vi "PWM Config.vi"(8 "error in (no error)":errorcluster, 11 "Config in":refnum<class "Config.lvclass">) -> (0 "error out":errorcluster, 1 "IDs found?":bool, 2 "PWM Data":T1, 3 "Config out":refnum<class "Config.lvclass">, 5 "File Found?":bool)   [LabVIEW 2019, in "Config.lvlib" / "Config.lvclass"]
doc: "Use this VI to retrieve the PWM channels that will be used in the robot."
uses:
  Config.lvclass
  Controls/PWM Data.ctl
  <vilib>/Rock Robotics/SystemInterfaces/DIO/FPGA_DIOPWMChannel.ctl
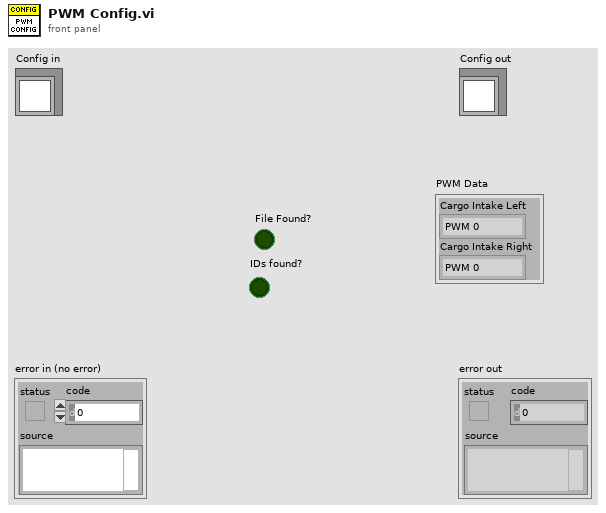
[diagram p1: front panel]
types:
  T1 = typedef "Config.lvlib/Config.lvclass/PWM Data.ctl" = cluster{"Cargo Intake Left":T2, "Cargo Intake Right":T2}
  T2 = typedef "FPGA_DIOPWMChannel.ctl" = enum8{"PWM 0", "PWM 1", "PWM 2", "PWM 3", "PWM 4", "PWM 5", "PWM 6", "PWM 7", "PWM 8", "PWM 9", "PWM MXP 0", "PWM MXP 1", "PWM MXP 2", "PWM MXP 3", "PWM MXP 4", "PWM MXP 5", "PWM MXP 6", "PWM MXP 7", "PWM MXP 8", "PWM MXP 9", "Invalid"}
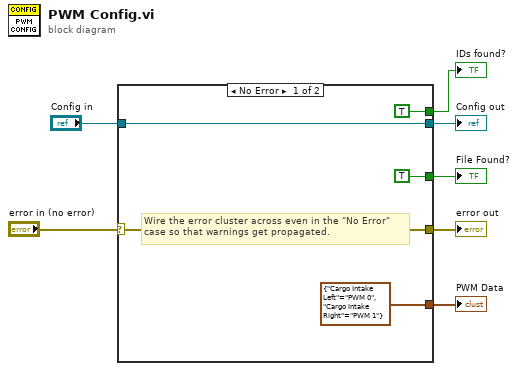
[diagram p0: block diagram]
diagram:
  n1 = case shown="No Error" "error in (no error)" {
    selector: "error in (no error)" -> [w11 w14]
    tunnel: [w11 w14] -> w6
    tunnel: [w12 w13] -> w4
    tunnel: "Config in" -> [w12 w13]
    tunnel: [TRUE ("IDs found?") _] -> w3
    tunnel: [TRUE ("File Found?") _] -> w2
    tunnel: [T1 {"Cargo Intake Left"=enum."PWM 0", "Cargo Intake Right"=enum."PWM 1"} ("PWM Data") _] -> w1
    frame No Error {
      # "Wire the error cluster across even in the \"No Error\"\ncase so that warnings get propagated."
    }
    frame Error {
    }
  }
  "error out" <- w6
  "Config out" <- w4
  "File Found?" <- w2
  "IDs found?" <- w3
  "PWM Data" <- w1
